vi "HandleDataSendError.vi"(7 "error info":string, 8 "error in (no error)":errorcluster, 9 "error code":i32, 10 "data send in":T1={"SendFileMode"=enum."Stream", "data"=variant, "InProgress"=FALSE}, 11 "Qbus in":refnum<class "Qbus.lvclass">) -> (0 "error out":errorcluster, 2 "data send out":T1={"SendFileMode"=enum."Stream", "data"=variant, "InProgress"=FALSE}, 3 "Qbus out":refnum<class "Qbus.lvclass">)   [LabVIEW 2017, in "ServerComm.lvlib"]
uses:
  <vilib>/addons/InsightCM/Devices/Shared/Common/ServerComm/ServerComm.lvlib
  <vilib>/addons/InsightCM/Devices/Shared/Common/ServerComm/controls/DataSendStatus.ctl
  <vilib>/addons/InsightCM/Devices/Shared/Common/ServerComm/controls/DataSendMode.ctl
  <vilib>/addons/Qbus/Qbus.lvclass
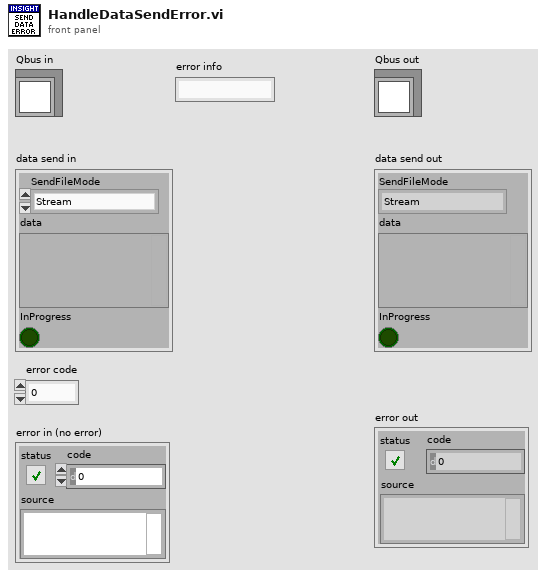
[diagram p1: front panel]
types:
  T1 = typedef "ServerComm.lvlib/DataSendStatus.ctl" = cluster{"SendFileMode":T2, "data":variant, "InProgress":bool}
  T2 = typedef "ServerComm.lvlib/DataSendMode.ctl" = enum16{"File", "InMemoryFile", "Stream", "StreamFileBlock", "ByteArray", "NoOp", "UnknownData"}
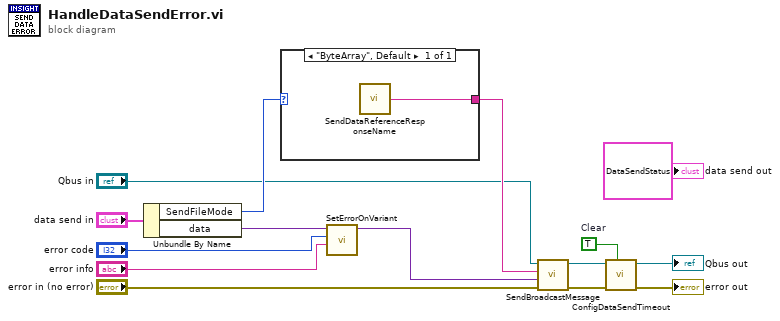
[diagram p0: block diagram]
diagram:
  w13 = TRUE  # Clear
  n1 = Unbundle By Name("data send in") -> ("SendFileMode"=w12:T2, "data"=w4:variant)
  n2 = case shown="\"ByteArray\", Default" w12 {
    tunnel: [w16] -> w11
    frame "ByteArray", Default {
      n3 = call <vilib>:"SendDataReferenceResponseName.vi"() -> ("message name"=w16:string)  [unwired: 5 in]
    }
  }
  n4 = call <vilib>:"SetErrorOnVariant.vi"("error info"="error info", "error code"="error code", "body in"=w4) -> ("body out"=w3:variant)  [unwired: 8 in]
  n5 = call <vilib>:"SendBroadcastMessage.vi"("error in (no error)"="error in (no error)", "message value"=w3, "message name"=w11, "Qbus in"="Qbus in") -> ("error in (no error)"=w15:errorcluster, "Qbus out"=w14:refnum<class "Qbus.lvclass">)  [unwired: 6 in]
  n6 = call <vilib>:"ConfigDataSendTimeout.vi"("clear"=w13, "error in (no error)"=w15, "Qbus in"=w14) -> ("error out"=→"error out":errorcluster, "Qbus out"=→"Qbus out":refnum<class "Qbus.lvclass">)  [unwired: 7 in]
  "data send out" <- T1 {"SendFileMode"=enum."Stream", "data"=variant, "InProgress"=FALSE} ("DataSend out")
